vi "Practica 8 Tejada ITIW31.vi"() -> ()   [LabVIEW 2018]
panel:
  out "Watts":dbl
  in  "Frecuencia HZ":dbl
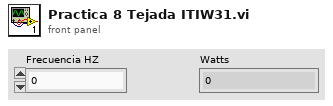
[diagram p1: front panel]
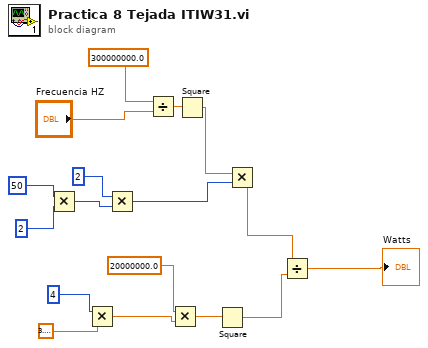
[diagram p0: block diagram]
diagram:
  n1 = Multiply(x=50, y=2) -> (x*y=w15:i32)
  n2 = Multiply(x=4, y=3.141592653589793) -> (x*y=w11:dbl)
  n3 = Multiply(x=2, y=w15) -> (x*y=w6:i32)
  n4 = Divide(x=300000000.0, y="Frecuencia HZ") -> (x/y=w7:dbl)
  n5 = Multiply(x=20000000.0, y=w11) -> (x*y=w4:dbl)
  n6 = Square(x=w7) -> (x^2=w5:dbl)
  n7 = Square(x=w4) -> (x^2=w2:dbl)
  n8 = Multiply(x=w5, y=w6) -> (x*y=w3:dbl)
  n9 = Divide(x=w3, y=w2) -> (x/y=→"Watts":dbl)
